vi "Set Property.vi"(8 "error in (no error)":errorcluster, 10 "Numeric":dbl, 11 "Test Class 1 in":refnum<class "Test Class 1.lvclass">) -> (0 "error out":errorcluster, 2 "Meter":dbl(knob) scale=0.0..10.0, 3 "Test Class 1 out":refnum<class "Test Class 1.lvclass">)   [LabVIEW 2024, in "Test Class 1.lvclass"]
uses:
  Test Class 1.lvclass
  Test Class 1.lvclass/Test Class 1.ctl
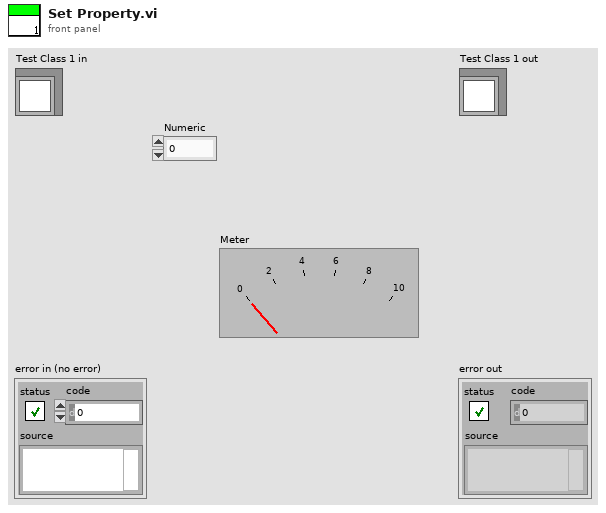
[diagram p1: front panel]
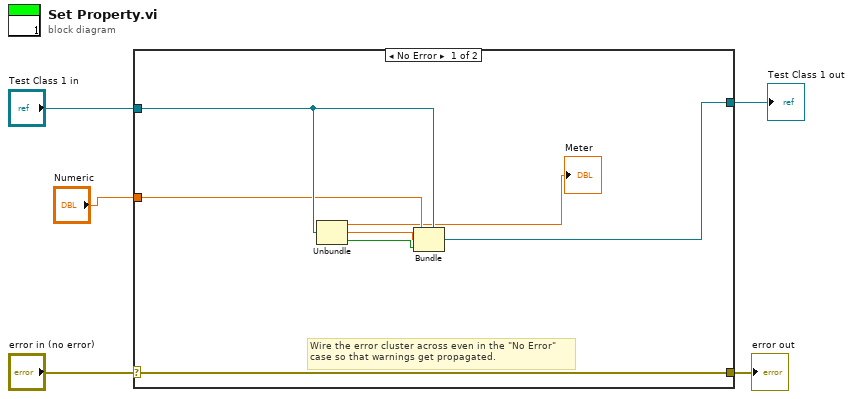
[diagram p0: block diagram]
diagram:
  n1 = case shown="No Error" "error in (no error)" {
    selector: "error in (no error)" -> [w12 w14]
    tunnel: [w12 w14] -> w4
    tunnel: "Test Class 1 in" -> [w11 w13]
    tunnel: [w10 w13] -> w2
    tunnel: "Numeric" -> [w7 _]
    frame No Error {
      # "Wire the error cluster across even in the \"No Error\"\ncase so that warnings get propagated."
      n2 = Unbundle(w11) -> (→"Meter":dbl, w9:dbl, w8:bool)
      n3 = Bundle(cluster=w11, w7, w9, w8) -> (w10:refnum<class "Test Class 1.lvclass">)
    }
    frame Error {
    }
  }
  "error out" <- w4
  "Test Class 1 out" <- w2
